vi "ROI 그리기.vi"(8 "ROI_Y":i32=200, 9 "ROI_X":i32=200, 11 "도형형태":u16(ring) items=["정사각형ROI", "삼각형ROI"]) -> (0 "Y좌표":i32[](array[numeric]), 3 "X좌표":i32[](array[numeric]))   [LabVIEW 2019]
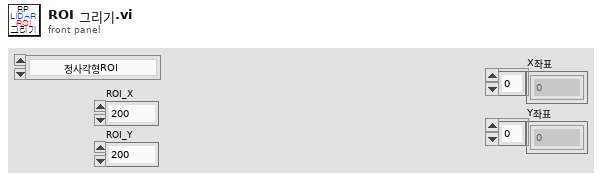
[diagram p1: front panel]
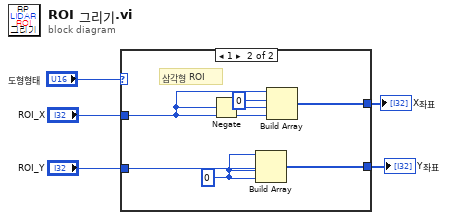
[diagram p0: block diagram]
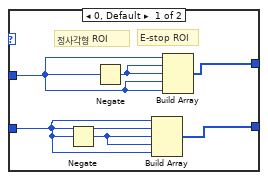
[diagram p2: hidden frame]
diagram:
  n1 = case shown="1" "도형형태" {
    tunnel: [w11 w15] -> w2
    tunnel: [w10 w14] -> w1
    tunnel: "ROI_X" -> [w7 w13]
    tunnel: "ROI_Y" -> [w6 w12]
    frame 0, Default {
      # "E-stop ROI"
      # "정사각형 ROI"
      n2 = Negate(x=w6) -> (-x=w8:i32)
      n3 = Negate(x=w7) -> (-x=w9:i32)
      n4 = Build Array(w6, w6, w8, w8, w6) -> (w10:i32[])
      n5 = Build Array(w7, w9, w9, w7, w7) -> (w11:i32[])
    }
    frame 1 {
      w17 = 0 ("element")
      # "삼각형 ROI"
      n6 = Negate(x=w13) -> (-x=w18:i32)
      n7 = Build Array(w17, w12, w17, w17) -> (w14:i32[])
      n8 = Build Array(w13, 0 ("element"), w18, w13) -> (w15:i32[])
    }
  }
  "X좌표" <- w2
  "Y좌표" <- w1
